vi "observacao.vi"() -> ()   [LabVIEW 2012] (continued)
                        n2689 = case shown="False" w3511 {
                          tunnel: [20 w3523] -> w3514
                          tunnel: w3513 -> [w3517 _]
                          tunnel: w3512 -> [_ _]
                          frame False {
                            w3521 = u16 2 items=["ZERO", "AH", "DEC", "TUBO", "CUP"] ("Controlador")
                            # "CLP Pronto"
                            n2690 = local write "DEC on Target"(FALSE ("DEC on Target")) -> ()
                            n2691 = call "rad_hms.vi"("TRUE=HORA\nFALSE=GRAU"=FALSE, "Radiano"=w3517) -> ("Hora/Graus Texto Decimal"=w3518:string)  [unwired: 3 in]
                            n2692 = call "Monta Comando.vi"("Set Point"=w3518, "Comando"="MOVER_RAP", "Dispositivo"="EIXO" ("Comando"), "Controlador"=w3521) -> ()  [unwired: 3 in, 3 out]
                          }
                          frame True {
                            # "CLP Ocupado"
                            n2693 = local read "TimeoutDEC 2"() -> (w3525:u32)
                            n2694 = call "TickTimeout.vi"("msInicial"=w3525, "msTimeout"=u32 4000) -> ("Timeout"=w3524:bool)  [unwired: 2 out]
                            n2695 = case shown="False" w3524 {
                              tunnel: [1 5] -> w3523
                              frame False {
                              }
                              frame True {
                                # "Tratar\nTimeout"
                              }
                            }
                          }
                        }
                      }
                      frame True {
                        # "Dist. pequena p/ mov. rápido"
                        # "Ligar mov. lento"
                        n2696 = call "TickTimeout.vi"() -> ("msTick"=w3529:u32)  [unwired: 2 in, 2 out]
                        n2697 = local write "TimeoutDEC 2"(w3529) -> ()
                      }
                    }
                    n2698 = local write "dec="(FALSE ("dec=")) -> ()
                  }
                  frame 2 {
                    w3537 = u16 12 items=["Alarme", "Atencao", "Erro", "Ocupado", "Protecao", "Embreagem", "Tracking", "Var. Track", "Rápido", "Ligeiro", "Médio", "Lento", "Em movimento", ""] ("NomeStatus")
                    # "Aguarda fim mov. Rap."
                    n2699 = call "Bit Status DEC.vi"("NomeStatus"=w3537) -> ("StatBit"=w3538:bool)
                    n2700 = case shown="True" w3538 {
                      tunnel: [1 w3547] -> w3535
                      tunnel: w3531 -> [_ w3546]
                      frame False {
                        # "Motor parado.\nTestar se chegou\nao destino"
                        n2701 = call "TickTimeout.vi"() -> ("msTick"=w3543:u32)  [unwired: 2 in, 2 out]
                        n2702 = local write "TimeoutDEC 2"(w3543) -> ()
                      }
                      frame True {
                        # "Ainda movendo...\nAGUARDAR"
                        n2703 = call "PROTECAO_DEC_UTILS.vi"("Destino DEC"=w3546) -> ("CONT DEC"=w3545:i32)  [unwired: 10 in]
                        n2704 = local read "Erro PROTEC"() -> (w3548:i32)
                        n2705 = Greater Or Equal?(x=w3545, y=w3548) -> (x >= y?=w3551:bool)
                        n2706 = local write "CONT DEC UTILS"(w3545) -> ()
                        n2707 = Select(t=6, s=w3551, f=2) -> (s? t:f=w3547:i32)
                      }
                    }
                    n2708 = global read "Global_Telescopio.vi" "Habilita supervisao"() -> (w3533:bool)
                    n2709 = case shown="True" w3533 {
                      tunnel: [FALSE w3542] -> w3532
                      frame False {
                      }
                      frame True {
                        n2710 = local read "CR DEC UTILS"() -> (w3540:i32)
                        n2711 = local read "Erro Lim"() -> (w3541:i32)
                        n2712 = Greater Or Equal?(x=w3540, y=w3541) -> (x >= y?=w3542:bool)
                      }
                    }
                    n2713 = Select(t=6, s=w3532, f=w3535) -> (s? t:f=w3534:i32)
                  }
                  frame 3 {
                    # "Mov.Lento"
                    n2714 = Subtract(x=w3553, y=w3556) -> (x-y=w3554:dbl)
                    n2715 = Absolute Value(x=w3554) -> (abs(x)=w3558:dbl)
                    n2716 = Less Or Equal?(x=w3558, y=w3557) -> (x <= y?=w3555:bool)
                    n2717 = case shown="False" w3555 {
                      tunnel: [w3561 0] -> w3559
                      tunnel: w3554 -> [w3560 _]
                      tunnel: w3552 -> [w3562 _]
                      frame False {
                        n2718 = case shown="False" w3562 {
                          tunnel: [40 w3571] -> w3561
                          tunnel: w3560 -> [w3565 _]
                          frame False {
                            w3570 = u16 2 items=["ZERO", "AH", "DEC", "TUBO", "CUP"] ("Controlador")
                            # "Mov. lento"
                            n2719 = call "TickTimeout.vi"() -> ("msTick"=w3563:u32)  [unwired: 2 in, 2 out]
                            n2720 = local write "TimeoutDEC 2"(w3563) -> ()
                            n2721 = call "rad_hms.vi"("TRUE=HORA\nFALSE=GRAU"=FALSE ("TRUE=HORA\nFALSE=GRAU"), "Radiano"=w3565) -> ("Hora/Graus Texto Decimal"=w3567:string)  [unwired: 3 in]
                            n2722 = call "Monta Comando.vi"("Set Point"=w3567, "Comando"="MOVER_REL", "Dispositivo"="EIXO" ("Comando"), "Controlador"=w3570) -> ()  [unwired: 3 in, 3 out]
                          }
                          frame True {
                            # "CLP Ocupado"
                            n2723 = local read "TimeoutDEC 2"() -> (w3573:u32)
                            n2724 = call "TickTimeout.vi"("msInicial"=w3573, "msTimeout"=u32 2000) -> ("Timeout"=w3572:bool)  [unwired: 2 out]
                            n2725 = case shown="False" w3572 {
                              tunnel: [3 5] -> w3571
                              frame False {
                              }
                              frame True {
                              }
                            }
                          }
                        }
                      }
                      frame True {
                        # "DEC no destino"
                        n2726 = local write "DEC on Target"(TRUE ("DEC on Target")) -> ()
                      }
                    }
                  }
                  frame 4 {
                    w3585 = u16 12 items=["Alarme", "Atencao", "Erro", "Ocupado", "Protecao", "Embreagem", "Tracking", "Var. Track", "Rápido", "Ligeiro", "Médio", "Lento", "Em movimento", ""] ("NomeStatus")
                    # "Aguarda fim mov. lento"
                    n2727 = call "Bit Status DEC.vi"("NomeStatus"=w3585) -> ("StatBit"=w3586:bool)
                    n2728 = case shown="True" w3586 {
                      tunnel: [3 w3596] -> w3581
                      tunnel: w3579 -> [_ w3594]
                      frame False {
                        # "Motor parado.\nTestar se chegou\nao destino"
                        n2729 = call "TickTimeout.vi"() -> ("msTick"=w3591:u32)  [unwired: 2 in, 2 out]
                        n2730 = local write "TimeoutDEC 2"(w3591) -> ()
                      }
                      frame True {
                        n2731 = call "PROTECAO_DEC_UTILS.vi"("Destino DEC"=w3594) -> ("CONT DEC"=w3593:i32)  [unwired: 10 in]
                        n2732 = local read "Erro PROTEC"() -> (w3599:i32)
                        n2733 = local write "CONT DEC UTILS"(w3593) -> ()
                        n2734 = Greater Or Equal?(x=w3593, y=w3599) -> (x >= y?=w3601:bool)
                        n2735 = local read "TimeoutDEC 2"() -> (w3595:u32)
                        n2736 = call "TickTimeout.vi"("msInicial"=w3595, "msTimeout"=u32 4000) -> ("Timeout"=w3598:bool)  [unwired: 2 out]
                        n2737 = case shown="False" w3598 {
                          tunnel: [4 5] -> w3602
                          frame False {
                          }
                          frame True {
                          }
                        }
                        n2738 = Select(t=6, s=w3601, f=w3602) -> (s? t:f=w3596:i32)
                      }
                    }
                    n2739 = global read "Global_Telescopio.vi" "Habilita supervisao"() -> (w3584:bool)
                    n2740 = case shown="True" w3584 {
                      tunnel: [FALSE w3590] -> w3580
                      frame False {
                      }
                      frame True {
                        n2741 = local read "CR DEC UTILS"() -> (w3588:i32)
                        n2742 = local read "Erro Lim"() -> (w3589:i32)
                        n2743 = Greater Or Equal?(x=w3588, y=w3589) -> (x >= y?=w3590:bool)
                      }
                    }
                    n2744 = Select(t=6, s=w3580, f=w3581) -> (s? t:f=w3582:i32)
                  }
                  frame 5 {
                    w3612 = u16 2 items=["ZERO", "AH", "DEC", "TUBO", "CUP"] ("Controlador")
                    # "Reiniciar apontamento"
                    # "Trata Timeout"
                    n2745 = call "TickTimeout.vi"() -> ("msTick"=w3605:u32)  [unwired: 2 in, 2 out]
                    n2746 = local write "TimeoutDEC 2"(w3605) -> ()
                    n2747 = call "Monta Comando.vi"("Comando"="PARAR", "Dispositivo"="PROG" ("Comando"), "Controlador"=w3612) -> ("Erro Comunicação"=w3607:bool)  [unwired: 4 in, 2 out]
                    n2748 = Select(t=6, s=w3607, f=1) -> (s? t:f=w3606:i32)
                  }
                  frame 6 {
                    n2749 = stacked-sequence {
                      frame #0 {
                        w3617 = u16 2 items=["ZERO", "AH", "DEC", "TUBO", "CUP"] ("Controlador")
                        # "Trata Timeout"
                        n2750 = local write "dec="(TRUE ("dec=")) -> ()
                        n2751 = call "Monta Comando.vi"("Comando"="PARAR", "Dispositivo"="PROG" ("Comando"), "Controlador"=w3617) -> ()  [unwired: 4 in, 3 out]
                      }
                      frame #1 {
                        w3619 = "Erro de Controlador DEC , REAPONTAR !" ("Mensagem")
                        n2752 = local write "Flag de erro p/ apagar lampada"(TRUE ("Flag de erro p/ apagar lampada")) -> ()
                        n2753 = call "Monta_Mensagem.vi"("Mensagem"=w3619) -> ()  [unwired: 2 in]
                        n2754 = call "Salva_systems_messages.vi"("Mensagem"=w3619) -> ()  [unwired: 5 in]
                      }
                      frame #2 {
                        w3621 = u16 2 items=["ZERO", "AH", "DEC", "TUBO", "CUP"] ("Controlador")
                        # "Em movimento não aceita reset"
                        # "Segundo PARAR por garantia"
                        n2755 = call "Monta Comando.vi"("Comando"="PARAR", "Dispositivo"="PROG", "Controlador"=w3621) -> ()  [unwired: 4 in, 3 out]
                      }
                    }
                  }
                  frame 20 {
                    # "Espera entrar\nem movimento"
                    n2756 = local read "Flag ativo DEC"() -> (w3624:bool)
                    n2757 = case shown="True" w3624 {
                      tunnel: [20 ("t") 2 ("t")] -> w3623
                      frame False {
                      }
                      frame True {
                        # "limpa flag"
                        n2758 = local write "Flag ativo DEC"(FALSE ("Flag ativo AH")) -> ()
                      }
                    }
                  }
                  frame 40 {
                    # "Espera entrar\nem movimento"
                    n2759 = local read "Flag ativo DEC"() -> (w3629:bool)
                    n2760 = case shown="True" w3629 {
                      tunnel: [40 ("t") 4 ("t")] -> w3628
                      frame False {
                      }
                      frame True {
                        # "limpa flag"
                        n2761 = local write "Flag ativo DEC"(FALSE ("Flag ativo AH")) -> ()
                      }
                    }
                  }
                }
                n2762 = case shown="1" "M_AH" {
                  selector: "M_AH" -> [w3635 _ _ _ _ _ _ _ _ _ _]
                  tunnel: [w3635 w3636 w3656 w3687 5 w3710 w3739 w3761 0 w3779 w3784] -> w3383
                  tunnel: "DestAH" -> [_ _ w3653 w3683 _ w3706 w3735 _ _ _ _]
                  tunnel: w3404 -> [_ _ w3659 _ _ w3712 _ _ _ _ _]
                  tunnel: w3399 -> [_ _ _ _ _ w3711 _ _ _ _ _]
                  tunnel: w3402 -> [_ _ w3660 _ _ _ _ _ _ _ _]
                  tunnel: w3397 -> [_ w3637 w3654 _ _ w3708 _ _ _ _ _]
                  frame 0, Default {
                    w3633 = 0 ("CR AH")
                    # "Sem apontamento"
                    n2763 = call "TickTimeout.vi"() -> ("msTick"=→"TimeoutAH 2":u32)  [unwired: 2 in, 2 out]
                    "CR AH UTILS" <- w3633
                    "CONT AH UTILS" <- w3633
                  }
                  frame 1 {
                    n2764 = case shown="False" w3637 {
                      tunnel: [2 w3647] -> w3636
                      frame False {
                        n2765 = stacked-sequence {
                          frame #0 {
                            w3642 = u16 1 items=["ZERO", "AH", "DEC", "TUBO", "CUP"] ("Controlador")
                            # "Desliga Acomp Sideral"
                            n2766 = call "Monta Comando.vi"("Comando"="DESLIGAR", "Dispositivo"="SIDERAL" ("Comando"), "Controlador"=w3642) -> ()  [unwired: 4 in, 3 out]
                          }
                          frame #1 {
                            w3645 = u16 1 items=["ZERO", "AH", "DEC", "TUBO", "CUP"] ("Controlador")
                            # "Parar Eixo AH"
                            n2767 = call "Monta Comando.vi"("Comando"="PARAR", "Dispositivo"="PROG" ("Comando"), "Controlador"=w3645) -> ()  [unwired: 4 in, 3 out]
                          }
                        }
                        n2768 = call "TickTimeout.vi"() -> ("msTick"=w3638:u32)  [unwired: 2 in, 2 out]
                        n2769 = local write "TimeoutAH 2"(w3638) -> ()
                      }
                      frame True {
                        n2770 = local read "TimeoutAH 2"() -> (w3646:u32)
                        n2771 = call "TickTimeout.vi"("msInicial"=w3646, "msTimeout"=u32 5000) -> ("Timeout"=w3649:bool)  [unwired: 2 out]
                        n2772 = case shown="False" w3649 {
                          tunnel: [1 7] -> w3647
                          frame False {
                          }
                          frame True {
                          }
                        }
                      }
                    }
                  }
                  frame 2 {
                    # "Mov.Rapido"
                    n2773 = Subtract(x=w3653, y=w3659) -> (x-y=w3657:dbl)
                    n2774 = Absolute Value(x=w3657) -> (abs(x)=w3658:dbl)
                    n2775 = Less?(x=w3658, y=w3660) -> (x < y?=w3655:bool)
                    n2776 = case shown="False" w3655 {
                      tunnel: w3653 -> [w3661 _]
                      tunnel: w3657 -> [_ _]
                      tunnel: [w3662 4] -> w3656
                      tunnel: w3654 -> [w3663 _]
                      frame False {
                        n2777 = case shown="False" w3663 {
                          tunnel: w3661 -> [w3669 _]
                          tunnel: [w3664 w3675] -> w3662
                          frame False {
                            w3671 = u16 1 items=["ZERO", "AH", "DEC", "TUBO", "CUP"] ("Controlador")
                            # "Aguardar\nfim mov."
                            # "Mov. rápido"
                            n2778 = local write "RA on Target"(FALSE ("RA on Target")) -> ()
                            n2779 = call "rad_hms.vi"("TRUE=HORA\nFALSE=GRAU"=TRUE ("TRUE=HORA\nFALSE=GRAU"), "Radiano"=w3669) -> ("Hora/Graus Texto Decimal"=w3674:string)  [unwired: 3 in]
                            n2780 = call "Monta Comando.vi"("Set Point"=w3674, "Comando"="MOVER_RAP", "Dispositivo"="EIXO" ("Comando"), "Controlador"=w3671) -> ("Erro Comunicação"=w3665:bool)  [unwired: 3 in, 2 out]
                            n2781 = Select(t=8, s=w3665, f=30) -> (s? t:f=w3664:i32)
                          }
                          frame True {
                            # "CLP Ocupado"
                            n2782 = local read "TimeoutAH 2"() -> (w3677:u32)
                            n2783 = call "TickTimeout.vi"("msInicial"=w3677, "msTimeout"=u32 4000) -> ("Timeout"=w3676:bool)  [unwired: 2 out]
                            n2784 = case shown="True" w3676 {
                              tunnel: [2 7] -> w3675
                              frame False {
                              }
                              frame True {
                                # "Tratar\nTimeout"
                              }
                            }
                          }
                        }
                      }
                      frame True {
                        # "Dist. pequena p/ mov. rápido"
                        n2785 = call "TickTimeout.vi"() -> ("msTick"=w3681:u32)  [unwired: 2 in, 2 out]
                        n2786 = local write "TimeoutAH 2"(w3681) -> ()
                      }
                    }
                    n2787 = local write "ah="(FALSE ("ah=")) -> ()
                  }
                  frame 3 {
                    w3690 = u16 12 items=["Alarme", "Atencao", "Erro", "Ocupado", "Protecao", "Embreagem", "Tracking", "Var. Track", "Rápido", "Ligeiro", "Médio", "Lento", "Em movimento", ""] ("NomeStatus")
                    # "Aguarda fim mov. Rap."
                    n2788 = call "Bit Status AH.vi"("NomeStatus"=w3690) -> ("StatBit"=w3689:bool)
                    n2789 = case shown="True" w3689 {
                      tunnel: [2 w3699] -> w3686
                      tunnel: w3683 -> [_ w3698]
                      frame False {
                        # "Motor parado.\nTestar se precisa\nde novo cmd. \nde mov. rápido"
                        n2790 = call "TickTimeout.vi"() -> ("msTick"=w3695:u32)  [unwired: 2 in, 2 out]
                        n2791 = local write "TimeoutAH 2"(w3695) -> ()
                      }
                      frame True {
                        # "Aqui também \ncaberia um \nTimeout?"
                        # "Ainda movendo...\nAGUARDAR"
                        n2792 = call "PROTECAO_AH_UTILS.vi"("DestinoAH"=w3698) -> ("CONT AH"=w3697:i32)  [unwired: 10 in]
                        n2793 = local read "Erro PROTEC"() -> (w3701:i32)
                        n2794 = local write "CONT AH UTILS"(w3697) -> ()
                        n2795 = Greater Or Equal?(x=w3697, y=w3701) -> (x >= y?=w3702:bool)
                        n2796 = Select(t=8, s=w3702, f=3) -> (s? t:f=w3699:i32)
                      }
                    }
                    n2797 = global read "Global_Telescopio.vi" "Habilita supervisao"() -> (w3685:bool)
                    n2798 = case shown="True" w3685 {
                      tunnel: [FALSE w3694] -> w3684
                      frame False {
                      }
                      frame True {
                        n2799 = local read "Erro Lim"() -> (w3693:i32)
                        n2800 = local read "CR AH UTILS"() -> (w3692:i32)
                        n2801 = Greater Or Equal?(x=w3692, y=w3693) -> (x >= y?=w3694:bool)
                      }
                    }
                    n2802 = Select(t=8, s=w3684, f=w3686) -> (s? t:f=w3687:i32)
                  }
                  frame 4 {
                    # "Não faz nada"
                    n2803 = call "TickTimeout.vi"() -> ("msTick"=w3705:u32)  [unwired: 2 in, 2 out]
                    n2804 = local write "TimeoutAH 2"(w3705) -> ()
                  }
                  frame 5 {
                    # "Mov.Lento"
                    n2805 = Subtract(x=w3706, y=w3712) -> (x-y=w3707:dbl)
                    n2806 = Absolute Value(x=w3707) -> (abs(x)=w3713:dbl)
                    n2807 = Less Or Equal?(x=w3713, y=w3711) -> (x <= y?=w3709:bool)
                    n2808 = case shown="True" w3709 {
                      tunnel: w3707 -> [w3715 _]
                      tunnel: [w3714 0] -> w3710
                      tunnel: w3708 -> [w3716 _]
                      frame False {
                        n2809 = case shown="False" w3716 {
                          tunnel: w3715 -> [w3721 _]
                          tunnel: [w3720 w3727] -> w3714
                          frame False {
                            w3723 = u16 1 items=["ZERO", "AH", "DEC", "TUBO", "CUP"] ("Controlador")
                            # "Envia Cmd. Mov. Lento"
                            n2810 = call "rad_hms.vi"("TRUE=HORA\nFALSE=GRAU"=TRUE ("TRUE=HORA\nFALSE=GRAU"), "Radiano"=w3721) -> ("Hora/Graus Texto Decimal"=w3726:string)  [unwired: 3 in]
                            n2811 = call "Monta Comando.vi"("Set Point"=w3726, "Comando"="MOVER_REL", "Dispositivo"="EIXO" ("Comando"), "Controlador"=w3723) -> ("Erro Comunicação"=w3718:bool)  [unwired: 3 in, 2 out]
                            n2812 = Select(t=8, s=w3718, f=60) -> (s? t:f=w3720:i32)
                          }
                          frame True {
                            # "CLP Ocupado"
                            n2813 = local read "TimeoutAH 2"() -> (w3729:u32)
                            n2814 = call "TickTimeout.vi"("msInicial"=w3729, "msTimeout"=u32 4000) -> ("Timeout"=w3728:bool)  [unwired: 2 out]
                            n2815 = case shown="False" w3728 {
                              tunnel: [5 7] -> w3727
                              frame False {
                              }
                              frame True {
                              }
                            }
                          }
                        }
                      }
                      frame True {
                        # "AH on Target"
                        n2816 = local write "RA on Target"(TRUE ("RA on Target")) -> ()
                      }
                    }
                  }
                  frame 6 {
                    w3742 = u16 12 items=["Alarme", "Atencao", "Erro", "Ocupado", "Protecao", "Embreagem", "Tracking", "Var. Track", "Rápido", "Ligeiro", "Médio", "Lento", "Em movimento", ""] ("NomeStatus")
                    # "Aguarda fim mov. Lento"
                    n2817 = call "Bit Status AH.vi"("NomeStatus"=w3742) -> ("StatBit"=w3741:bool)
                    n2818 = case shown="True" w3741 {
                      tunnel: [5 w3756] -> w3738
                      tunnel: w3735 -> [_ w3750]
                      frame False {
                        # "Motor parado.\nTestar se chegou\nao destino"
                        n2819 = call "TickTimeout.vi"() -> ("msTick"=w3747:u32)  [unwired: 2 in, 2 out]
                        n2820 = local write "TimeoutAH 2"(w3747) -> ()
                      }
                      frame True {
                        n2821 = local read "Erro PROTEC"() -> (w3758:i32)
                        n2822 = call "PROTECAO_AH_UTILS.vi"("DestinoAH"=w3750) -> ("CONT AH"=w3749:i32)  [unwired: 10 in]
                        n2823 = local write "CONT AH UTILS"(w3749) -> ()
                        n2824 = local read "TimeoutAH 2"() -> (w3751:u32)
                        n2825 = Greater Or Equal?(x=w3749, y=w3758) -> (x >= y?=w3752:bool)
                        n2826 = call "TickTimeout.vi"("msInicial"=w3751, "msTimeout"=u32 4000) -> ("Timeout"=w3755:bool)  [unwired: 2 out]
                        n2827 = case shown="False" w3755 {
                          tunnel: [6 7] -> w3753
                          frame False {
                          }
                          frame True {
                            # "Tratar\nTimeout"
                          }
                        }
                        n2828 = Select(t=8, s=w3752, f=w3753) -> (s? t:f=w3756:i32)
                      }
                    }
                    n2829 = global read "Global_Telescopio.vi" "Habilita supervisao"() -> (w3737:bool)
                    n2830 = case shown="True" w3737 {
                      tunnel: [FALSE w3746] -> w3736
                      frame False {
                      }
                      frame True {
                        n2831 = local read "CR AH UTILS"() -> (w3744:i32)
                        n2832 = local read "Erro Lim"() -> (w3745:i32)
                        n2833 = Greater Or Equal?(x=w3744, y=w3745) -> (x >= y?=w3746:bool)
                      }
                    }
                    n2834 = Select(t=8, s=w3736, f=w3738) -> (s? t:f=w3739:i32)
                  }
                  frame 7 {
                    w3766 = u16 1 items=["ZERO", "AH", "DEC", "TUBO", "CUP"] ("Controlador")
                    # "Reiniciar apontamento"
                    # "Trata Timeout"
                    n2835 = call "TickTimeout.vi"() -> ("msTick"=w3765:u32)  [unwired: 2 in, 2 out]
                    n2836 = local write "TimeoutAH 2"(w3765) -> ()
                    n2837 = call "Monta Comando.vi"("Comando"="PARAR", "Dispositivo"="PROG" ("Comando"), "Controlador"=w3766) -> ("Erro Comunicação"=w3762:bool)  [unwired: 4 in, 2 out]
                    n2838 = Select(t=8, s=w3762, f=2) -> (s? t:f=w3761:i32)
                  }
                  frame 8 {
                    n2839 = stacked-sequence {
                      frame #0 {
                        w3771 = u16 1 items=["ZERO", "AH", "DEC", "TUBO", "CUP"] ("Controlador")
                        # "Reiniciar apontamento"
                        # "Trata Timeout"
                        n2840 = local write "ah="(TRUE ("ah=")) -> ()
                        n2841 = call "Monta Comando.vi"("Comando"="PARAR", "Dispositivo"="PROG" ("Comando"), "Controlador"=w3771) -> ()  [unwired: 4 in, 3 out]
                      }
                      frame #1 {
                        w3775 = "Erro de Controlador RA , REAPONTAR !" ("Mensagem")
                        n2842 = local write "Flag de erro p/ apagar lampada"(TRUE ("Flag de erro p/ apagar lampada")) -> ()
                        n2843 = call "Monta_Mensagem.vi"("Mensagem"=w3775) -> ()  [unwired: 2 in]
                        n2844 = call "Salva_systems_messages.vi"("Mensagem"=w3775) -> ()  [unwired: 5 in]
                      }
                      frame #2 {
                        w3778 = u16 1 items=["ZERO", "AH", "DEC", "TUBO", "CUP"] ("Controlador")
                        # "Em movimento não aceita reset"
                        # "Segundo PARAR por garantia"
                        n2845 = call "Monta Comando.vi"("Comando"="PARAR", "Dispositivo"="PROG", "Controlador"=w3778) -> ()  [unwired: 4 in, 3 out]
                      }
                    }
                  }
                  frame 30 {
                    # "Espera entrar\nem movimento"
                    n2846 = local read "Flag ativo AH"() -> (w3780:bool)
                    n2847 = case shown="True" w3780 {
                      tunnel: [30 ("t") 3 ("t")] -> w3779
                      frame False {
                      }
                      frame True {
                        # "limpa flag"
                        n2848 = local write "Flag ativo AH"(FALSE ("Flag ativo AH")) -> ()
                      }
                    }
                  }
                  frame 60 {
                    # "Espera entrar\nem movimento"
                    n2849 = local read "Flag ativo AH"() -> (w3785:bool)
                    n2850 = case shown="True" w3785 {
                      tunnel: [60 ("t") 6 ("t")] -> w3784
                      frame False {
                      }
                      frame True {
                        # "limpa flag"
                        n2851 = local write "Flag ativo AH"(FALSE ("Flag ativo AH")) -> ()
                      }
                    }
                  }
                }
                n2852 = call "PROTECAO.vi"("Estado In"=w3381) -> ("Estado Out"=w3380:i32)  [unwired: 2 in]
                n2853 = call "PROTECAO.vi"("Estado In"=w3383) -> ("Estado Out"=w3382:i32)  [unwired: 2 in]
                n2854 = local write "M_DEC"(w3380) -> ()
                n2855 = property on="Setup, Pointing & Guiding" class="TabCtl (strict)"() -> ("Page Selector Visible"=w3387:bool)  [unwired: 2 in, 2 out]
                n2856 = local write "M_AH"(w3382) -> ()
                n2857 = global read "Global_Telescopio.vi" "PosCUP"() -> (w3395:i16)
                n2858 = global read "Global_Telescopio.vi" "ErroMaxCup"() -> (w3394:i16)
                n2859 = local read "M_PROT"() -> (w3377:i32)
                n2860 = call "Bit Status CUP.vi"("NomeStatus"=w3392) -> ("StatBit"=w3396:bool)
                n2861 = Not(x=w3387) -> (.not. x?=w3385:bool)
                n2862 = case shown="5" "M_CUP" {
                  selector: "M_CUP" -> [w3409 _ _ _ _ _ _ _ _]
                  tunnel: [w3409 w3410 w3441 1 w3453 w3470 w3475 w3492 0 ("estadoCUP")] -> w3379
                  tunnel: w3396 -> [_ w3412 _ _ w3452 _ w3476 _ _]
                  tunnel: w3395 -> [_ w3416 _ _ _ _ _ _ _]
                  tunnel: "DestCUP" -> [_ w3411 _ _ _ _ _ _ _]
                  tunnel: w3394 -> [_ w3414 _ _ _ _ _ _ _]
                  frame 0, Default {
                    # "Sem movimento"
                    n2863 = call "TickTimeout.vi"() -> ("msTick"=→"TimeoutCUP 2":u32)  [unwired: 2 in, 2 out]
                  }
                  frame 1 {
                    # "Envia\nComando"
                    n2864 = Subtract(x=w3411, y=w3416) -> (x-y=w3415:i16)
                    n2865 = Absolute Value(x=w3415) -> (abs(x)=w3417:i16)
                    n2866 = Less Or Equal?(x=w3417, y=w3414) -> (x <= y?=w3413:bool)
                    n2867 = case shown="True" w3413 {
                      tunnel: w3412 -> [w3420 _]
                      tunnel: w3411 -> [w3419 _]
                      tunnel: [w3418 w3435] -> w3410
                      frame False {
                        # "CUP fora pos."
                        n2868 = case shown="True" w3420 {
                          tunnel: w3419 -> [w3428 _]
                          tunnel: [2 w3429] -> w3418
                          frame False {
                            w3423 = u16 4 items=["ZERO", "AH", "DEC", "TUBO", "CUP"] ("Controlador")
                            # "CLP Pronto"
                            n2869 = Number To Decimal String(number=w3428) -> (decimal integer string=w3427:string)  [unwired: 1 in]
                            n2870 = call "TickTimeout.vi"() -> ("msTick"=w3422:u32)  [unwired: 2 in, 2 out]
                            n2871 = local write "Dome on Target"(FALSE ("Dome on Target")) -> ()
                            n2872 = local write "TimeoutCUP 2"(w3422) -> ()
                            n2873 = call "Monta Comando.vi"("Set Point"=w3427, "Comando"="MOVER", "Dispositivo"="DOMO" ("Comando"), "Controlador"=w3423) -> ()  [unwired: 3 in, 3 out]
                          }
                          frame True {
                            # "CLP Busy"
                            n2874 = local read "TimeoutCUP 2"() -> (w3431:u32)
                            n2875 = call "TickTimeout.vi"("msInicial"=w3431, "msTimeout"=u32 5000) -> ("Timeout"=w3430:bool)  [unwired: 2 out]
                            n2876 = case shown="True" w3430 {
                              tunnel: [1 3] -> w3429
                              frame False {
                              }
                              frame True {
                              }
                            }
                          }
                        }
                      }
                      frame True {
                        # "Verifica\nTrapeira e\nParavento"
                        # "CUP no destino"
                        n2877 = global read "Global_Telescopio.vi" "Parking"() -> (w3438:bool)
                        n2878 = call "TickTimeout.vi"() -> ("msTick"=w3439:u32)  [unwired: 2 in, 2 out]
                        n2879 = local write "TimeoutCUP 2"(w3439) -> ()
                        n2880 = Select(t=4, s=w3438, f=8) -> (s? t:f=w3435:i32)
                      }
                    }
                  }
                  frame 2 {
                    w3440 = u16 12 items=["Alarme", "Atencao", "Erro", "Ocupado", "TBD", "LCB", "Trapeira", "Paravento", "DomoRap", "DomoCW", "DomoCCW", "TBD", "Em movimento", "TBD"] ("NomeStatus")
                    # "Aqui também caberia um Timeout?"
                    # "Aguarda parada motor"
                    n2881 = call "Bit Status CUP.vi"("NomeStatus"=w3440) -> ("StatBit"=w3442:bool)
                    n2882 = case shown="False" w3442 {
                      tunnel: [1 2] -> w3441
                      frame False {
                        # "Motor parado.\nTestar se chegou\nao destino"
                        n2883 = call "TickTimeout.vi"() -> ("msTick"=w3443:u32)  [unwired: 2 in, 2 out]
                        n2884 = local write "TimeoutCUP 2"(w3443) -> ()
                      }
                      frame True {
                        # "Ainda movendo...\nAGUARDAR"
                      }
                    }
                  }
                  frame 3 {
                    w3449 = u16 4 items=["ZERO", "AH", "DEC", "TUBO", "CUP"] ("Controlador")
                    # "Trata Timeout"
                    n2885 = call "TickTimeout.vi"() -> ("msTick"=w3446:u32)  [unwired: 2 in, 2 out]
                    n2886 = local write "TimeoutCUP 2"(w3446) -> ()
                    n2887 = call "Monta Comando.vi"("Comando"="PARAR", "Dispositivo"="PROG" ("Comando"), "Controlador"=w3449) -> ()  [unwired: 4 in, 3 out]
                  }
                  frame 4 {
                    # "Verifica Trapeira"
                    n2888 = case shown="True" "Case Constant\n(See Context Help) 13" {
                      tunnel: [4 w3455] -> w3453
                      tunnel: w3452 -> [_ w3456]
                      frame False {
                      }
                      frame True {
                        n2889 = case shown="False" w3456 {
                          tunnel: [5 w3461] -> w3455
                          frame False {
                            w3460 = u16 4 items=["ZERO", "AH", "DEC", "TUBO", "CUP"] ("Controlador")
                            # "Fechar Trapeira"
                            # "Aguardar abertura Trap."
                            # "CLP Pronto"
                            n2890 = call "Monta Comando.vi"("Comando"="FECHAR", "Dispositivo"="TRAPEIRA" ("Comando"), "Controlador"=w3460) -> ()  [unwired: 4 in, 3 out]
                          }
                          frame True {
                            # "CLP Busy"
                            n2891 = local read "TimeoutCUP 2"() -> (w3463:u32)
                            n2892 = call "TickTimeout.vi"("msInicial"=w3463, "msTimeout"=u32 5000) -> ("Timeout"=w3462:bool)  [unwired: 2 out]
                            n2893 = case shown="False" w3462 {
                              tunnel: [4 3] -> w3461
                              frame False {
                              }
                              frame True {
                              }
                            }
                          }
                        }
                      }
                    }
                  }
                  frame 5 {
                    w3468 = u16 6 items=["Alarme", "Atencao", "Erro", "Ocupado", "TBD", "LCB", "Trapeira", "Paravento", "DomoRap", "DomoCW", "DomoCCW", "TBD", "Em movimento", "TBD"] ("NomeStatus")
                    # "Aqui também caberia um Timeout?"
                    # "Aguarda Fechamento da Trapeira"
                    # "Também poderia ser testado o bit \"Em movimento\".\nNeste caso o código do \"IF\" deve ser permutado."
                    n2894 = call "Bit Status CUP.vi"("NomeStatus"=w3468) -> ("StatBit"=w3469:bool)
                    n2895 = Not(x=w3469) -> (.not. x?=w3467:bool)
                    n2896 = case shown="True" w3467 {
                      tunnel: [5 6] -> w3470
                      frame False {
                        # "Ainda movendo...\nAGUARDAR"
                      }
                      frame True {
                        # "Trapeira Fechada.\nVerificar Paravento."
                        n2897 = call "TickTimeout.vi"() -> ("msTick"=w3472:u32)  [unwired: 2 in, 2 out]
                        n2898 = local write "TimeoutCUP 2"(w3472) -> ()
                      }
                    }
                  }
                  frame 6 {
                    # "Verifica Paravento"
                    n2899 = case shown="True" "Case Constant\n(See Context Help) 14" {
                      tunnel: w3476 -> [_ w3479]
                      tunnel: [8 w3478] -> w3475
                      frame False {
                        # "Paravento Elevado"
                      }
                      frame True {
                        # "Subir Parav."
                        n2900 = case shown="False" w3479 {
                          tunnel: [7 w3484] -> w3478
                          frame False {
                            w3483 = u16 4 items=["ZERO", "AH", "DEC", "TUBO", "CUP"] ("Controlador")
                            # "Aguardar subida Parav."
                            # "CLP Pronto"
                            n2901 = call "Monta Comando.vi"("Comando"="SUBIR", "Dispositivo"="PARAVENTO" ("Comando"), "Controlador"=w3483) -> ()  [unwired: 4 in, 3 out]
                          }
                          frame True {
                            # "CLP Busy"
                            n2902 = local read "TimeoutCUP 2"() -> (w3486:u32)
                            n2903 = call "TickTimeout.vi"("msInicial"=w3486, "msTimeout"=u32 5000) -> ("Timeout"=w3485:bool)  [unwired: 2 out]
                            n2904 = case shown="False" w3485 {
                              tunnel: [6 3] -> w3484
                              frame False {
                              }
                              frame True {
                              }
                            }
                          }
                        }
                      }
                    }
                  }
                  frame 7 {
                    w3491 = u16 7 items=["Alarme", "Atencao", "Erro", "Ocupado", "TBD", "LCB", "Trapeira", "Paravento", "DomoRap", "DomoCW", "DomoCCW", "TBD", "Em movimento", "TBD"] ("NomeStatus")
                    # "Também poderia ser testado o bit \"Em movimento\".\nNeste caso o código do \"IF\" deve ser permutado."
                    # "Aguarda Subida Paravento"
                    n2905 = call "Bit Status CUP.vi"("NomeStatus"=w3491) -> ("StatBit"=w3493:bool)
                    n2906 = Not(x=w3493) -> (.not. x?=w3490:bool)
                    n2907 = case shown="False" w3490 {
                      tunnel: [7 8] -> w3492
                      frame False {
                        # "Ainda movendo...\nAGUARDAR"
                      }
                      frame True {
                        # "Paravento elevado."
                      }
                    }
                  }
                  frame 8 {
                    # "CUP on target"
                    n2908 = local write "Dome on Target"(TRUE ("Dome on Target")) -> ()
                    n2909 = global write "Global_Telescopio.vi" "Parking"(FALSE) -> ()
                  }
                }
                n2910 = call "PROTECAO.vi"("Estado In"=w3379) -> ("Estado Out"=w3378:i32)  [unwired: 2 in]
                n2911 = Compound Arithmetic op=ADD(w3377, w3378, w3382, w3380) -> (w3388:i32)
                n2912 = Equal To 0?(x=w3388) -> (x = 0?=w3386:bool)
                n2913 = And(x=w3386, y=w3385) -> (x .and. y?=w3384:bool)
                n2914 = case shown="True" w3384 {
                  frame False {
                  }
                  frame True {
                    w3405 = FALSE
                    w3406 = u8 0 ("Disabled")
                    # "DESLIGA TODOS"
                    # "HABILITA TODOS"
                    n2915 = local write "BtUtilZenith"(w3405) -> ()
                    n2916 = local write "BtUtilPark"(w3405) -> ()
                    n2917 = local write "PROTEÇÃO"(w3405) -> ()
                    n2918 = local write "FLAT-FIELD"(w3405) -> ()
                    n2919 = local write "ECASS"(w3405) -> ()
                    n2920 = property on="BtUtilPark" class="Bool (strict)"("Disabled"=w3406) -> ()  [unwired: 2 in, 2 out]
                    n2921 = property on="ECASS" class="Bool (strict)"("Disabled"=w3406) -> ()  [unwired: 2 in, 2 out]
                    n2922 = property on="Setup, Pointing & Guiding" class="TabCtl (strict)"("Page Selector Visible"=TRUE) -> ()  [unwired: 2 in, 2 out]
                    n2923 = property on="BtUtilZenith" class="Bool (strict)"("Disabled"=w3406) -> ()  [unwired: 2 in, 2 out]
                    n2924 = property on="FLAT-FIELD" class="Bool (strict)"("Disabled"=w3406) -> ()  [unwired: 2 in, 2 out]
                    n2925 = property on="PROTEÇÃO" class="Bool (strict)"("Disabled"=w3406) -> ()  [unwired: 2 in, 2 out]
                  }
                }
                n2926 = local write "M_CUP"(w3378) -> ()
              }
              frame #4 {
                n2927 = case shown="True" "GO" {
                  frame False {
                  }
                  frame True {
                    w3793 = u16 3 items=["Alarme", "Atencao", "Erro", "Ocupado", "Protecao", "Embreagem", "Tracking", "Var. Track", "Rápido", "Ligeiro", "Médio", "Lento", "Em movimento", ""] ("NomeStatus")
                    w3794 = u16 3 items=["Alarme", "Atencao", "Erro", "Ocupado", "Protecao", "Embreagem", "Tracking", "Var. Track", "Rápido", "Ligeiro", "Médio", "Lento", "Em movimento", ""] ("NomeStatus")
                    n2928 = call "Bit Status AH.vi"("NomeStatus"=w3794) -> ("StatBit"=w3792:bool)
                    n2929 = call "Bit Status DEC.vi"("NomeStatus"=w3793) -> ("StatBit"=w3791:bool)
                    n2930 = Or(x=w3792, y=w3791) -> (x .or. y?=w3790:bool)
                    n2931 = case shown="False" w3790 {
                      frame False {
                        w3795 = FALSE ("RA on Target")
                        w3813 = u16 1 items=["ZERO", "AH", "DEC", "TUBO", "CUP"] ("Controlador")
                        w3818 = u16 2 items=["ZERO", "AH", "DEC", "TUBO", "CUP"] ("Controlador")
                        w3796 = FALSE ("GO")
                        n2932 = local write "RA on Target"(w3795) -> ()
                        n2933 = local write "DEC on Target"(w3795) -> ()
                        n2934 = global read "Global_Telescopio.vi" "Calagem AH"() -> (w3806:dbl)
                        n2935 = call "Comma_to_Point.vi"("Lat_A"="StrPointObjRA 2") -> ("Saída"=w3800:string)
                        n2936 = call "Comma_to_Point.vi"("Lat_A"="StrPointObjDEC 2") -> ("Saída"=w3797:string)
                        n2937 = global read "Global_Telescopio.vi" "Calagem DEC"() -> (w3805:dbl)
                        n2938 = call "hms_rad.vi"("True = hora"=TRUE, "Texto Graus"=w3800) -> ("radianos"=w3801:dbl)  [unwired: 3 in]
                        n2939 = call "hms_rad.vi"("True = hora"=FALSE, "Texto Graus"=w3797) -> ("radianos"=w3802:dbl)  [unwired: 3 in]
                        n2940 = Add(x=w3801, y=w3806) -> (x+y=w3804:dbl)
                        n2941 = Add(x=w3802, y=w3805) -> (x+y=w3803:dbl)
                        n2942 = local write "GO"(w3796) -> ()
                        n2943 = global write "Global_Telescopio.vi" "ObjCentrado"(w3796) -> ()
                        n2944 = call "rad_hms.vi"("TRUE=HORA\nFALSE=GRAU"=TRUE ("TRUE=HORA\nFALSE=GRAU"), "Radiano"=w3804) -> ("Hora/Graus Texto Decimal"=w3810:string)  [unwired: 3 in]
                        n2945 = call "rad_hms.vi"("TRUE=HORA\nFALSE=GRAU"=FALSE, "Radiano"=w3803) -> ("Hora/Graus Texto Decimal"=w3809:string)  [unwired: 3 in]
                        n2946 = call "Monta Comando.vi"("Set Point"=w3810, "Comando"="MOVER_ABS", "Dispositivo"="EIXO" ("Comando"), "Controlador"=w3813) -> ()  [unwired: 3 in, 3 out]
                        n2947 = call "Monta Comando.vi"("Set Point"=w3809, "Comando"="MOVER_ABS", "Dispositivo"="EIXO" ("Comando"), "Controlador"=w3818) -> ()  [unwired: 3 in, 3 out]
                      }
                      frame True {
                      }
                    }
                  }
                }
              }
            }
          }
        }
      }
      frame #3 {
        # "Desabiita Centragem\ndurante apontamento"
        # "PROCESSO TRACKING"
        # "Comando Via serial do Sist\nAquisição"
        # "CHAVES PAINEL"
        n2948 = local read "FLAT-FIELD"() -> (w3819:bool)
        n2949 = local read "BtUtilZenith"() -> (w3820:bool)
        n2950 = case shown="True" "BtShutterClose" {
          frame False {
          }
          frame True {
            w3864 = u16 3 items=["Alarme", "Atencao", "Erro", "Ocupado", "TBD", "LCB", "Trapeira", "Paravento", "DomoRap", "DomoCW", "DomoCCW", "TBD", "Em movimento", "TBD"] ("NomeStatus")
            n2951 = call "Bit Status CUP.vi"("NomeStatus"=w3864) -> ("StatBit"=w3865:bool)
            n2952 = case shown="False" w3865 {
              selector: w3865 -> [w3866 _]
              frame False {
                w3869 = u16 4 items=["ZERO", "AH", "DEC", "TUBO", "CUP"] ("Controlador")
                n2953 = local write "BtShutterClose"(w3866) -> ()
                n2954 = call "Monta Comando.vi"("Comando"="FECHAR", "Dispositivo"="TRAPEIRA" ("Comando"), "Controlador"=w3869) -> ()  [unwired: 4 in, 3 out]
              }
              frame True {
              }
            }
          }
        }
        n2955 = Or(x=w3820, y=w3819) -> (x .or. y?=w3821:bool)
        n2956 = case shown="True" w3821 {
          frame False {
            w3838 = u16 3 items=["Alarme", "Atencao", "Erro", "Ocupado", "Protecao", "Embreagem", "Tracking", "Var. Track", "Rápido", "Ligeiro", "Médio", "Lento", "Em movimento", ""] ("NomeStatus")
            n2957 = call "Bit Status AH.vi"("NomeStatus"=w3838) -> ("StatBit"=w3837:bool)
            n2958 = case shown="False" "MOUNT" {
              tunnel: w3837 -> [w3840 w3849]
              frame False {
                n2959 = local read "LED MOUNT"() -> (w3841:bool)
                n2960 = Not(x=w3840) -> (.not. x?=w3843:bool)
                n2961 = And(x=w3843, y=w3841) -> (x .and. y?=w3842:bool)
                n2962 = case shown="True" w3842 {
                  frame False {
                  }
                  frame True {
                    w3845 = FALSE
                    w3846 = u16 1 items=["ZERO", "AH", "DEC", "TUBO", "CUP"] ("Controlador")
                    n2963 = call "Monta Comando.vi"("Comando"="DESLIGAR", "Dispositivo"="SIDERAL" ("Comando"), "Controlador"=w3846) -> ()  [unwired: 4 in, 3 out]
                    n2964 = local write "LED MOUNT"(w3845) -> ()
                    n2965 = global write "Global_Telescopio.vi" "ObjCentrado"(w3845) -> ()
                    n2966 = property on="Calagem" class="Bool"("Disabled"=u8 2) -> ()  [unwired: 2 in, 2 out]
                  }
                }
              }
              frame True {
                n2967 = local read "LED MOUNT"() -> (w3850:bool)
                n2968 = Or(x=w3849, y=w3850) -> (x .or. y?=w3851:bool)
                n2969 = case shown="False" w3851 {
                  frame False {
                    w3852 = u16 1 items=["ZERO", "AH", "DEC", "TUBO", "CUP"] ("Controlador")
                    n2970 = call "Monta Comando.vi"("Comando"="LIGAR", "Dispositivo"="SIDERAL" ("Comando"), "Controlador"=w3852) -> ()  [unwired: 4 in, 3 out]
                    "LED MOUNT" <- TRUE
                  }
                  frame True {
                  }
                }
              }
            }
          }
          frame True {
            n2971 = local write "LED MOUNT"(FALSE) -> ()
          }
        }
        n2972 = case shown="True" "Stop All" {
          frame False {
          }
          frame True {
            # "MUDANÇA:\nDesligada chave do\nacompanhamento."
            n2973 = local write "MOUNT"(FALSE ("Led Start/Stop")) -> ()
            n2974 = global write "Global_Telescopio.vi" "STOP ALL"(TRUE ("STOP ALL")) -> ()
          }
        }
        n2975 = case shown="True" "RESTART METEOR" {
          frame False {
          }
          frame True {
            n2976 = call "Teste_Read_Meteorologica.vi"() -> ("Erro"=w3870:bool)  [unwired: 2 in]
            n2977 = local write "Default Met"(w3870) -> ()
          }
        }
        n2978 = global read "Global_Telescopio.vi" "Centragem Via Aquisicao"() -> (w3834:bool)
        n2979 = case shown="True" "STOP" {
          frame False {
          }
          frame True {
            n2980 = stacked-sequence {
              frame #0 {
                n2981 = call "Stop.vi"() -> ()  [unwired: 1 in, 1 out]
              }
              frame #1 {
                w3857 = 0 ("estado")
                n2982 = local write "statDEC"(w3857) -> ()
                n2983 = local write "statAH"(w3857) -> ()
                n2984 = local write "statCUP"(w3857) -> ()
              }
              frame #2 {
                w3858 = 0 ("estado")
                n2985 = local write "M_AH"(w3858) -> ()
                n2986 = local write "M_DEC"(w3858) -> ()
                n2987 = local write "M_CUP"(w3858) -> ()
                n2988 = local write "M_PROT"(w3858) -> ()
              }
              frame #3 {
                n2989 = case shown="True" "Case Constant\n(See Context Help) 15" {
                  frame False {
                  }
                  frame True {
                    w3860 = FALSE
                    n2990 = local write "BtUtilZenith"(w3860) -> ()
                    n2991 = local write "FLAT-FIELD"(w3860) -> ()
                    n2992 = local write "PROTEÇÃO"(w3860) -> ()
                    n2993 = local write "BtUtilPark"(w3860) -> ()
                    n2994 = local write "ECASS"(w3860) -> ()
                  }
                }
              }
              frame #4 {
                n2995 = case shown="True" "LedPointing" {
                  frame False {
                  }
                  frame True {
                    n2996 = local write "LedPointing"(FALSE ("LedPointing")) -> ()
                    n2997 = global write "Global_Telescopio.vi" "Botão GO = STOP"(TRUE ("Botão GO = STOP")) -> ()
                  }
                }
              }
            }
          }
        }
        n2998 = control-ref of="BtTargetPoint"() -> (w3826:refnum<vi>)
        n2999 = And(x="Enable Centragem", y=w3834) -> (x .and. y?=w3833:bool)
        n3000 = property class="Bool"(reference=w3826) -> ("Boolean Text.Text"=w3827:string)  [unwired: 1 in, 2 out]
        n3001 = Or(x="BtOnTatget", y=w3833) -> (x .or. y?=w3829:bool)
        n3002 = Equal?(x=w3827, y="STOP") -> (x = y?=w3825:bool)
        n3003 = Not(x=w3825) -> (.not. x?=w3824:bool)
        n3004 = And(x=w3824, y=w3829) -> (x .and. y?=w3830:bool)
        n3005 = case shown="True" w3830 {
          frame False {
          }
          frame True {
            n3006 = stacked-sequence {
              seq-local: [w3871 _ _ _] -> [_ _ _ w3936]
              seq-local: [_ w3885 _ _] -> [_ _ _ w3937]
              seq-local: [_ _ w3899 _] -> [_ _ _ w3938]
              frame #0 {
                # "Transforma estados lógicos\nnuma string hexadecimal"
                n3007 = local read "Processa Centragem"() -> (w3875:bool)
                n3008 = local read "MOV_IDX_AH"() -> (w3873:bool)
                n3009 = local read "ChkModel"() -> (w3877:bool)
                n3010 = local read "MOV_IDX_DEC"() -> (w3872:bool)
                n3011 = global read "Global_Telescopio.vi" "CalLocal"() -> (w3879:bool)
                n3012 = global read "Global_Telescopio.vi" "CalGlobal"() -> (w3878:bool)
                n3013 = global read "Global_Telescopio.vi" "CoordDia"() -> (w3876:bool)
                n3014 = global read "Global_Telescopio.vi" "ObjCentrado"() -> (w3874:bool)
                n3015 = Build Array(w3879, w3878, w3877, w3876, w3875, w3874, w3873, w3872) -> (w3882:bool[])
                n3016 = Boolean Array To Number(Boolean array=w3882) -> (number=w3881:u32)
                n3017 = Number To Hexadecimal String(1:i16 2 ("width (-)"), 2:w3881) -> (0:w3871:string)
              }
              frame #1 {
                w3886 = "\t"
                # "Reseta Flag do comando oriundo\nda comunicação serial Aquisição"
                n3018 = local read "ChkPointPrecessed"() -> (w3883:bool)
                n3019 = local read "StrPointObjName"() -> (w3889:string)
                "NAME" <- w3889
                n3020 = local read "StrPointObjRA"() -> (w3888:string)
                "RA" <- w3888
                n3021 = local read "StrPointObjDEC"() -> (w3887:string)
                "DEC" <- w3887
                n3022 = case shown="True" w3883 {
                  tunnel: ["2000.0" ("Saída") w3893] -> w3884
                  frame False {
                  }
                  frame True {
                    n3023 = call "Calcula epoch.vi"() -> ("epoch"=w3896:dbl)  [unwired: 2 in]
                    n3024 = Number To Fractional String(number=w3896, precision (6)=i16 1) -> (F-format string=w3894:string)  [unwired: 2 in]
                    n3025 = call "Comma_to_Point.vi"("Lat_A"=w3894) -> ("Saída"=w3893:string)
                  }
                }
                n3026 = global write "Global_Telescopio.vi" "Centragem Via Aquisicao"(FALSE ("Centragem Via Aquisicao")) -> ()
                n3027 = local write "Processa Centragem"(TRUE) -> ()
                n3028 = global write "Global_Telescopio.vi" "NAME OBJETO"(w3889) -> ()
                n3029 = global write "Global_Telescopio.vi" "DEC AQUIS"(w3887) -> ()
                n3030 = global write "Global_Telescopio.vi" "RA AQUIS"(w3888) -> ()
                n3031 = Concatenate Strings(w3889, w3886, w3888, w3886, w3887) -> (w3885:string)
                n3032 = global write "Global_Telescopio.vi" "EPOCH AQUIS"(w3884) -> ()
              }
              frame #2 {
                w3897 = "\t"
                w3912 = FALSE ("use system decimal point (T)")
                w3913 = i16 1 ("precision (6)")
                n3033 = global read "Global_Telescopio.vi" "Right Ascention"() -> (w3903:string)
                n3034 = global read "Global_Telescopio.vi" "Calagem DEC"() -> (w3929:dbl)
                n3035 = global read "Global_Telescopio.vi" "Calagem AH"() -> (w3926:dbl)
                n3036 = global read "Global_Telescopio.vi" "Sideral Time"() -> (w3922:dbl)
                n3037 = global read "Global_Telescopio.vi" "Sideral time"() -> (w3900:string)
                n3038 = global read "Global_Telescopio.vi" "Hour Angle"() -> (w3901:string)
                n3039 = global read "Global_Telescopio.vi" "Declination"() -> (w3902:string)
                n3040 = global read "Global_Telescopio.vi" "TargetDEC"() -> (w3917:dbl)
                n3041 = local read "Offset DEC"() -> (w3915:dbl)
                n3042 = global read "Global_Telescopio.vi" "TargetRA"() -> (w3916:dbl)
                n3043 = local read "Offset RA"() -> (w3914:dbl)
                n3044 = global read "Global_Telescopio.vi" "PosDEC"() -> (w3920:dbl)
                n3045 = global read "Global_Telescopio.vi" "PosAH"() -> (w3923:dbl)
                n3046 = local read "UT"() -> (w3898:string)
                n3047 = Subtract(x=w3922, y=w3923) -> (x-y=w3921:dbl)
                n3048 = call "rad_hms.vi"("TRUE=HORA\nFALSE=GRAU"=TRUE ("TRUE=HORA\nFALSE=GRAU"), "Radiano"=w3916) -> ("Hora/Graus Texto Decimal"=w3910:string)  [unwired: 3 in]
                n3049 = call "rad_hms.vi"("TRUE=HORA\nFALSE=GRAU"=FALSE ("TRUE=HORA\nFALSE=GRAU"), "Radiano"=w3917) -> ("Hora/Graus Texto Decimal"=w3909:string)  [unwired: 3 in]
                n3050 = call "rad_hms.vi"("TRUE=HORA\nFALSE=GRAU"=TRUE ("TRUE=HORA\nFALSE=GRAU"), "Radiano"=w3921) -> ("Hora/Graus Texto Decimal"=w3908:string)  [unwired: 3 in]
                n3051 = call "rad_hms.vi"("TRUE=HORA\nFALSE=GRAU"=FALSE ("TRUE=HORA\nFALSE=GRAU"), "Radiano"=w3920) -> ("Hora/Graus Texto Decimal"=w3907:string)  [unwired: 3 in]
                n3052 = call "rad_hms.vi"("TRUE=HORA\nFALSE=GRAU"=TRUE, "Radiano"=w3926) -> ("Hora/Graus Texto Decimal"=w3906:string)  [unwired: 3 in]
                n3053 = call "rad_hms.vi"("TRUE=HORA\nFALSE=GRAU"=FALSE, "Radiano"=w3929) -> ("Hora/Graus Texto Decimal"=w3911:string)  [unwired: 3 in]
                n3054 = Number To Fractional String(use system decimal point (T)=w3912, number=w3915, precision (6)=w3913) -> (F-format string=w3905:string)  [unwired: 1 in]
                n3055 = Number To Fractional String(use system decimal point (T)=w3912, number=w3914, precision (6)=w3913) -> (F-format string=w3904:string)  [unwired: 1 in]
                n3056 = Concatenate Strings(w3910, w3897, w3909, w3897, w3908, w3897, w3907, w3897, w3906, w3897, w3911, w3897, w3905, w3897, w3904, w3897, w3903, w3897, w3902, w3897, w3901, w3897, w3900, w3897, w3898) -> (w3899:string)
              }
              frame #3 {
                w3935 = "\t"
                # "Condições atmosféricas"
                # "Dados de catálogo do Objeto"
                # "Tempo e posição do telescópio"
                # "Estados das variáveis de processos"
                n3057 = global read "Global_Telescopio.vi" "Data Arq LOG"() -> (w3950:string)
                n3058 = local read "AtmosferaStr"() -> (w3933:string)
                n3059 = Concatenate Strings("C:\\TCS\\LOG\\AP_" ("SOMENTE DIRETORIO"), w3950, ".TXT" ("SOMENTE DIRETORIO")) -> (w3949:string)
                n3060 = String To Path(string=w3949) -> (path=w3948:path)
                n3061 = call <vilib>:"Open_Create_Replace File.vi"("function (open:0)"=T8."open or create", "file path"=w3948) -> ("error out"=w3945:errorcluster, "refnum"=w3946:refnum<file>)  [unwired: 6 in, 2 out]
                n3062 = Concatenate Strings(w3938, w3935, w3937, w3935, w3933, w3935, w3936, "\r\n") -> (w3939:string)
                n3063 = Set File Position(refnum=w3946, from (0:start)=enum16{"start", "end", "current"}."end" ("pos mode (0:2)"), error in=w3945) -> (refnum out=w3932:refnum<file>, error out=w3931:errorcluster)  [unwired: 1 in]
                n3064 = Write to Binary File(file (use dialog)=w3932, data=w3939, error in=w3931, 5:FALSE ("prepend array or string size? (T)")) -> (refnum out=w3942:refnum<file>, error out=w3943:errorcluster)  [unwired: 2 in, 1 out]
                n3065 = Close File(refnum=w3942, error in=w3943) -> (error out=w3941:errorcluster)  [unwired: 1 out]
                n3066 = call <vilib>:"Simple Error Handler.vi"("error in (no error)"=w3941) -> ()  [unwired: 4 in, 5 out]
              }
            }
          }
        }
      }
      frame #4 {
        # "Abre Imagens"
        # "ABAS DE IMAGENS"
        n3067 = case shown="\"Image 1\", Default" "Tab Control" {
          frame "Image 1", Default {
            n3068 = disable-structure shown="Disabled" {
              frame Disabled {
                # "Imagem oriunda do\nconector BNC 1"
                n3069 = global read "Global_Telescopio.vi" "Tempo Atulização Cam 0"() -> (w3960:i16)
                n3070 = call "timepulse_Cam_0.vi"("de quantos segundos"=w3960) -> ("PULSO"=w3963:bool)  [unwired: 2 in]
                n3071 = Or(x="IMAGE 5", y=w3963) -> (x .or. y?=w3962:bool)
                n3072 = case shown="True" w3962 {
                  frame False {
                  }
                  frame True {
                    n3073 = call "AngeloRTV_Snap.vi"("PortNo"=u16 0) -> ("depth"=w3969:u8, "color table"=w3967:u32[], "rect"=w3970:T11, "flattened image data"=w3968:u8[])  [unwired: 2 in, 1 out]
